vi "Configure Data Buffer.vi"(0 "VISA resource name":refnum<visa-resource-name>, 1 "Enable Buffer (F: Disable)":bool, 5 "Buffer Feed (0: Input Signal)":u16(ring) items=["Input Signal", "Math Result", "Relative Result"], 7 "Readings Buffered (100)":i32=100, 11 "error in (no error)":errorcluster) -> (4 "VISA resource name out":refnum<visa-resource-name>, 15 "error out":errorcluster)   [LabVIEW 2020, in "Keithley 648X Series.lvlib"]
doc: "Configures the data buffer feed, reading storage capacity, and enables or disables reading buffering."
uses:
  <instrlib>/Keithley 648X Series/Keithley 648X Series.lvlib
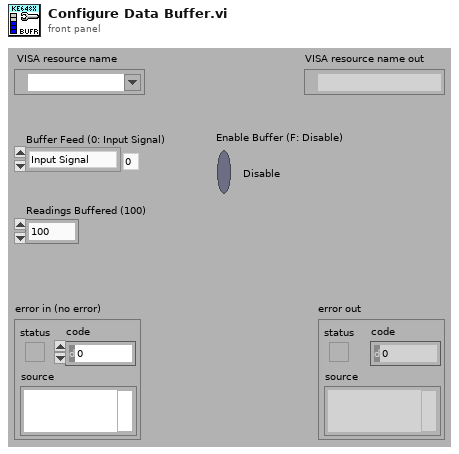
[diagram p1: front panel]
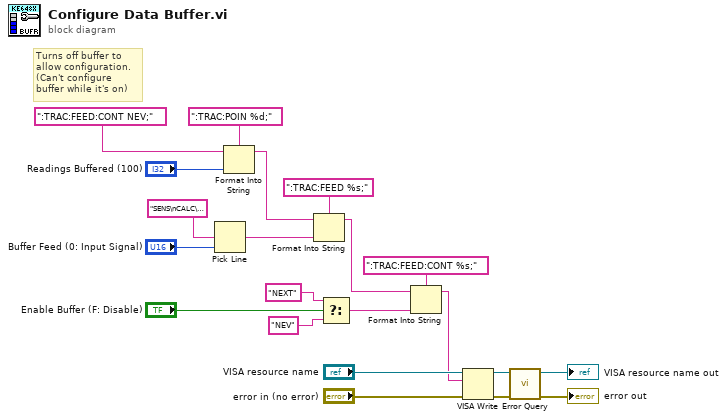
[diagram p0: block diagram]
diagram:
  # "Turns off buffer to\nallow configuration.\n(Can't configure\nbuffer while it's on)"
  n1 = Pick Line(multi-line string="SENS\nCALC\nCALC2", line index="Buffer Feed (0: Input Signal)") -> (output string=w9:string)  [unwired: 1 in]
  n2 = Format Into String(format string=":TRAC:POIN %d;", initial string=":TRAC:FEED:CONT NEV;", "Readings Buffered (100)") -> (resulting string=w13:string)  [unwired: 1 in, 1 out]
  n3 = Format Into String(format string=":TRAC:FEED %s;", initial string=w13, w9) -> (resulting string=w2:string)  [unwired: 1 in, 1 out]
  n4 = Select(t="NEXT" ("format string"), s="Enable Buffer (F: Disable)", f="NEV" ("format string")) -> (s? t:f=w4:string)
  n5 = Format Into String(format string=":TRAC:FEED:CONT %s;", initial string=w2, w4) -> (resulting string=w3:string)  [unwired: 1 in, 1 out]
  n6 = VISA Write(VISA resource name="VISA resource name", write buffer=w3, error in (no error)="error in (no error)") -> (VISA resource name out=w17:refnum<visa-resource-name>, error out=w16:errorcluster)  [unwired: 1 out]
  n7 = call <instrlib>:"Error Query.vi"("error in (no error)"=w16, "VISA resource name"=w17) -> ("error out"=→"error out":errorcluster, "VISA resource name out"=→"VISA resource name out":refnum<visa-resource-name>)  [unwired: 6 in, 2 out]
